vi "json_labview_2012.vi"(8 "error in":errorcluster, 11 "Path":path) -> (0 "error out":errorcluster, 3 "data from JSON file":T1)   [LabVIEW 2012]
panel:
  out "Expected format":string
  out "JSON file content":string
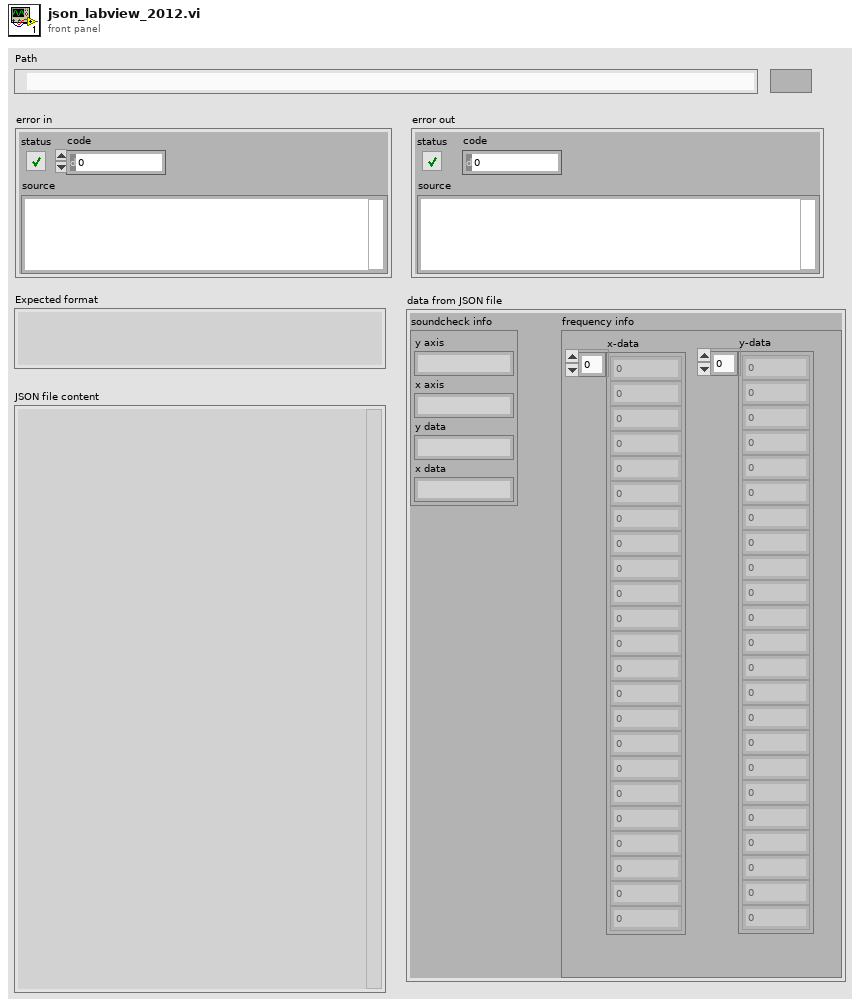
[diagram p1: front panel]
types:
  T1 = cluster{"frequency info":cluster{"y-data":dbl[], "x-data":dbl[]}, "soundcheck info":cluster{"y axis":string, "x axis":string, "y data":string, "x data":string}}
  T2 = enum16{"open", "replace", "create", "open or create", "replace or create", "replace or create with confirmation"}
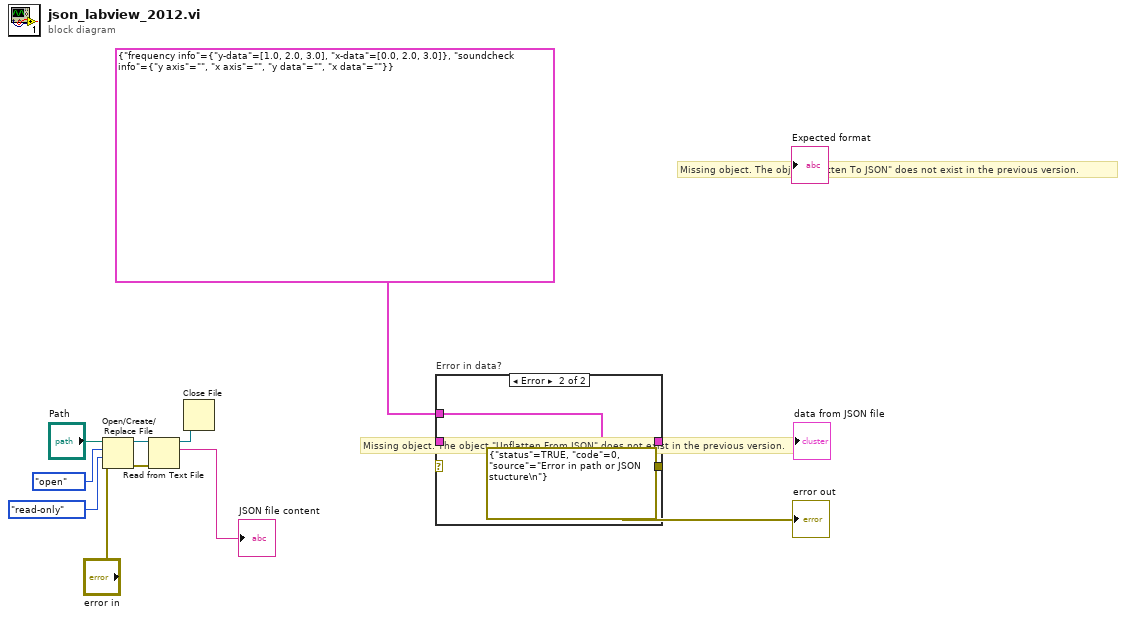
[diagram p0: block diagram]
diagram:
  # "Missing object. The object \"Unflatten From JSON\" does not exist in the previous version."
  # "Missing object. The object \"Flatten To JSON\" does not exist in the previous version."
  n1 = Open/Create/Replace File(file path (use dialog)="Path", error in="error in", operation (0:open)=T2."open", access (0:read/write)=enum16{"read/write", "read-only", "write-only"}."read-only") -> (refnum out=w12:refnum<file>, error out=w11:errorcluster)  [unwired: 2 in, 1 out]
  n2 = Read from Text File(file (use dialog)=w12, error in=w11) -> (refnum out=w10:refnum<file>, text=→"JSON file content":string, error out=w7:errorcluster)  [unwired: 2 in, 1 out]
  n3 = Close File(refnum=w10) -> ()  [unwired: 1 in, 2 out]
  n4 = case "Error in data?" shown="Error" w6 {
    selector: [w16 _] -> w6
    tunnel: [w17 w19] -> w5
    tunnel: [w17 _] -> w4
    tunnel: T1 {"frequency info"={"y-data"=[1.0, 2.0, 3.0], "x-data"=[0.0, 2.0, 3.0]}, "soundcheck info"={"y axis"="", "x axis"="", "y data"="", "x data"=""}} -> [_ w19]
    tunnel: [w16 errorcluster {"status"=TRUE, "code"=0, "source"="Error in path or JSON stucture\n"} ("error out")] -> w1
    frame No Error {
    }
    frame Error {
    }
  }
  "data from JSON file" <- w5
  "error out" <- w1
